vi "Phasor Compute Base Frequency & Harmonic Orders.vi"(8 "Error In":errorcluster, 11 "Frequency Array":dbl[](array[numeric])) -> (0 "Error Out":errorcluster, 1 "Harmonic Orders":i32[](array[numeric]), 3 "Base Frequency":dbl)   [LabVIEW 2021, in "Phasor.lvlib"]
uses:
  Phasor.lvlib
  Math/Math.lvlib
  <vilib>/gmath/NI_Gmath.lvlib
panel:
  out "D Array":u32[](array[numeric])
  out "N Array":i32[](array[numeric])
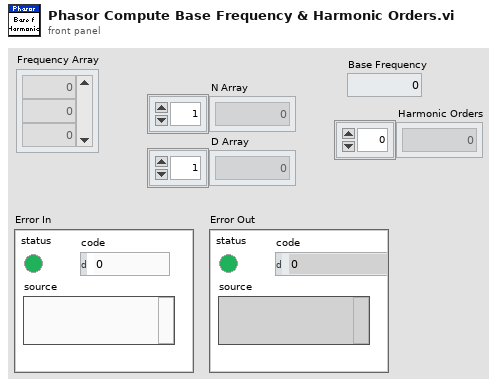
[diagram p1: front panel]
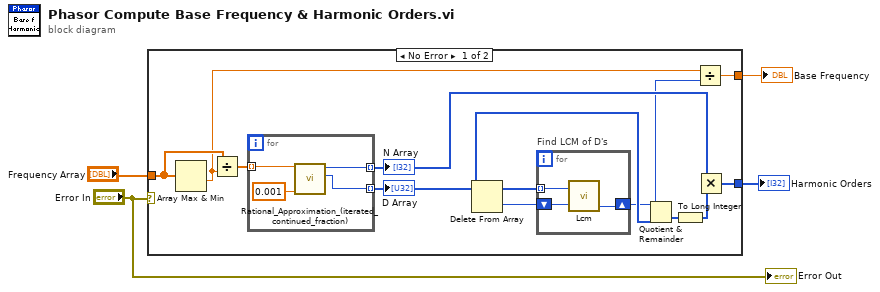
[diagram p0: block diagram]
diagram:
  n1 = case shown="No Error" "Error In" {
    tunnel: "Frequency Array" -> [w16 _]
    tunnel: [w10 _] -> w3
    tunnel: [w7 _] -> w2
    frame No Error {
      n2 = Array Max & Min(array=w16) -> (min value=w8:dbl)  [unwired: 3 out]
      n3 = Divide(x=w16, y=w8) -> (x/y=w15:dbl[])
      n4 = for {
        tunnel: w15 -> [w23] mode=indexing
        tunnel: [w21] -> w11 mode=indexing
        tunnel: [w20] -> w6 mode=indexing
        n5 = call "Rational_Approximation_(iterated_continued_fraction).vi"("tol (1.0e-6)"=0.001, "X"=w23) -> ("D: denominator"=w20:u32, "N: numerator"=w21:i32)  [unwired: 7 in, 1 out]
      }
      "N Array" <- w11
      "D Array" <- w6
      n6 = Delete From Array(array=w6) -> (deleted portion=w13:u32, array with subset deleted=w14:u32[])  [unwired: 2 in]
      n7 = for "Find LCM of D's" {
        tunnel: w14 -> [w18] mode=indexing
        shift-right: [w17] -> w5
        shift-left: w13 -> [w19]
        n8 = call <vilib>:"Lcm.vi"("y"=w19, "x"=w18) -> ("lcm(x,y)"=w17:i64)
      }
      n9 = Quotient & Remainder(x=w5, y=w6) -> (floor(x/y)=w12:i64[])  [unwired: 1 out]
      n10 = To Long Integer(number=w12) -> (32bit integer=w9:i32[])
      n11 = Divide(x=w8, y=w5) -> (x/y=w7:dbl)
      n12 = Multiply(x=w11, y=w9) -> (x*y=w10:i32[])
    }
    frame Error {
    }
  }
  "Harmonic Orders" <- w3
  "Base Frequency" <- w2
  "Error Out" <- "Error In"
